vi "test_ccd_acqCount.vi"(8 "error in":errorcluster, 11 "CCD in":refnum<class "CCD.lvclass">) -> (0 "error out":errorcluster, 3 "CCD out":refnum<class "CCD.lvclass">)   [LabVIEW 2020, in "horiba.test.lvlib"]
uses:
  horiba.test.lvlib
  Classes/CCD/CCD.lvclass
  <vilib>/addons/_JKI Toolkits/Caraya/classes/Assert/Assert Equal Value and Type_Variant.vi
  15e7fe39-3d4f-4ccc-ae5c-22e5f2c5c50b.vi
panel:
  # "Connector Pane"
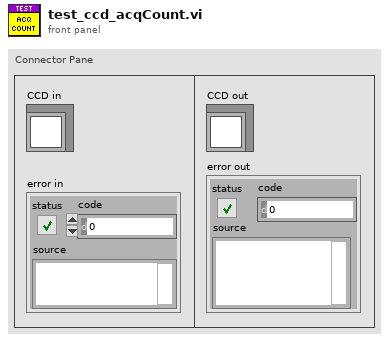
[diagram p1: front panel]
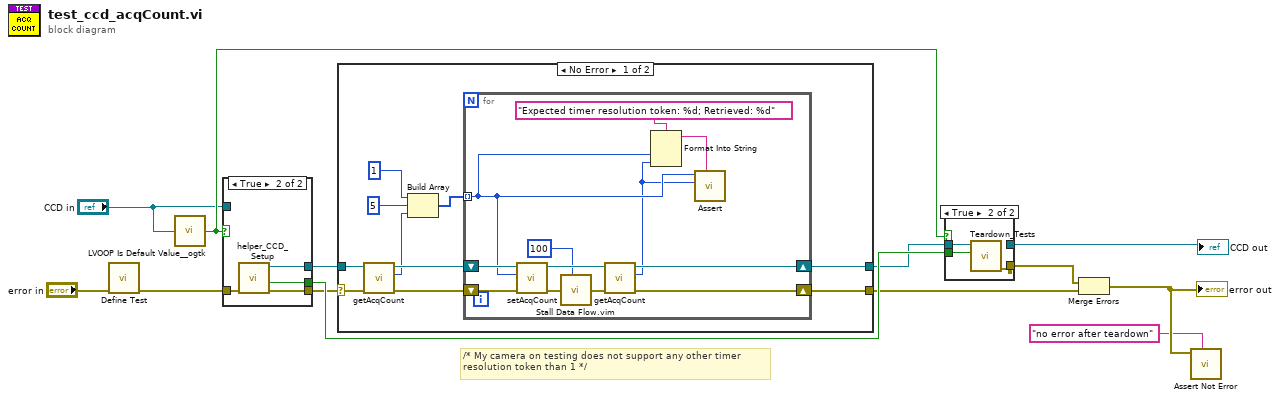
[diagram p0: block diagram]
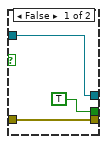
[diagram p3: hidden frame]
diagram:
  # "/* My camera on testing does not support any other timer \nresolution token than 1 */"
  n1 = call <vilib>:"Define Test.vi"("error in (no error)"="error in") -> ("error out"=w8:errorcluster)  [unwired: 9 in, 1 out]
  n2 = call <userlib>:"LVOOP Is Default Value__ogtk.vi"("Object"="CCD in") -> ("Is Default Value?"=w9:bool)
  n3 = case shown="True" w9 {
    tunnel: w8 -> [w15 w20]
    tunnel: [w15 w19] -> w4
    tunnel: [w16 w18] -> w6
    tunnel: [TRUE ("Module Was Already Running?") w17] -> w10
    tunnel: "CCD in" -> [w16 _]
    frame False {
    }
    frame True {
      n4 = call "helper_CCD_Setup.vi"("error in"=w20) -> ("error out"=w19:errorcluster, "Module Was Already Running?"=w17:bool, "CCD out"=w18:refnum<class "CCD.lvclass">)  [unwired: 7 in, 1 out]
    }
  }
  n5 = case shown="No Error" w4 {
    selector: w4 -> [w30 w43]
    tunnel: [w27 w44] -> w5
    tunnel: w6 -> [w29 w44]
    tunnel: [w25 w43] -> w3
    frame No Error {
      n6 = call "getAcqCount.vi"("error in (no error)"=w30, "CCD in"=w29) -> ("error out"=w26:errorcluster, "count"=w21:i32, "CCD out"=w28:refnum<class "CCD.lvclass">)  [unwired: 7 in]
      n7 = Build Array(1 ("token"), 5 ("element"), w21) -> (w23:i32[])
      n8 = for {
        shift-right: [w39] -> w27
        shift-left: w28 -> [w40]
        shift-right: [w37] -> w25
        shift-left: w26 -> [w38]
        tunnel: w23 -> [w34] mode=indexing
        n9 = call "setAcqCount.vi"("error in (no error)"=w38, "count"=w34, "CCD in"=w40) -> ("error out"=w42:errorcluster, "CCD out"=w41:refnum<class "CCD.lvclass">)  [unwired: 5 in, 2 out]
        n10 = call "Stall Data Flow.vim"("value in"=w42, "milliseconds to wait"=u32 100) -> ("value out"=w32:errorcluster)  [unwired: 1 out]
        n11 = call "getAcqCount.vi"("error in (no error)"=w32, "CCD in"=w41) -> ("error out"=w37:errorcluster, "count"=w33:i32, "CCD out"=w39:refnum<class "CCD.lvclass">)  [unwired: 7 in]
        n12 = Format Into String(format string="Expected timer resolution token: %d; Retrieved: %d", w34, w33) -> (resulting string=w36:string)  [unwired: 2 in, 1 out]
        n13 = call-poly <vilib>:"Assert.vi"("Label"=w36, "Y"=w33, "X"=w34) -> ()  [unwired: 7 in, 2 out]
      }
    }
    frame Error {
    }
  }
  n14 = case shown="True" w9 {
    tunnel: w5 -> [w45 w48]
    tunnel: [_ w47] -> w7
    tunnel: w10 -> [_ w46]
    tunnel: [w45 _] -> w1
    frame False {
    }
    frame True {
      n15 = call "Teardown_Tests.vi"("Module Was Already Running?"=w46, "horiba.lvlib:GenericDevice"=w48) -> ("error out"=w47:errorcluster)  [unwired: 8 in, 1 out]
    }
  }
  "CCD out" <- w1
  n16 = Merge Errors(w7, w3) -> (w12:errorcluster)
  "error out" <- w12
  n17 = call <vilib>:"Assert Not Error.vi"("Label"="no error after teardown", "Not Error?"=w12) -> ()  [unwired: 8 in, 2 out]
